vi "Write Non-Sequential Address.vi"(7 "Target IC (1-8)":u8, 8 "error in (no error)":errorcluster, 9 "Data":u16 format="%04x", 10 "Address":u16 format="%04x", 11 "FPGA Interface in":refnum<class "FPGA Interface.lvclass">) -> (0 "error out":errorcluster)   [LabVIEW 2020, in "BCI-1553 API.lvlib" / "FPGA Interface.lvlib" / "FPGA Interface.lvclass"]
doc: "Write a value to an arbitrary address on a component in the 1553 Session."
uses:
  FPGA Interface.lvclass
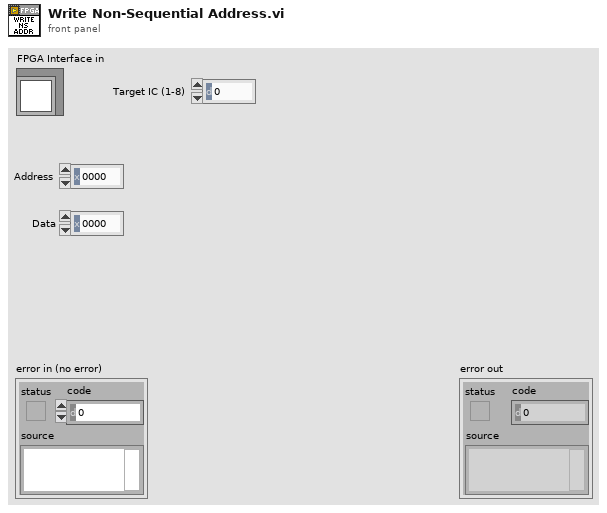
[diagram p1: front panel]
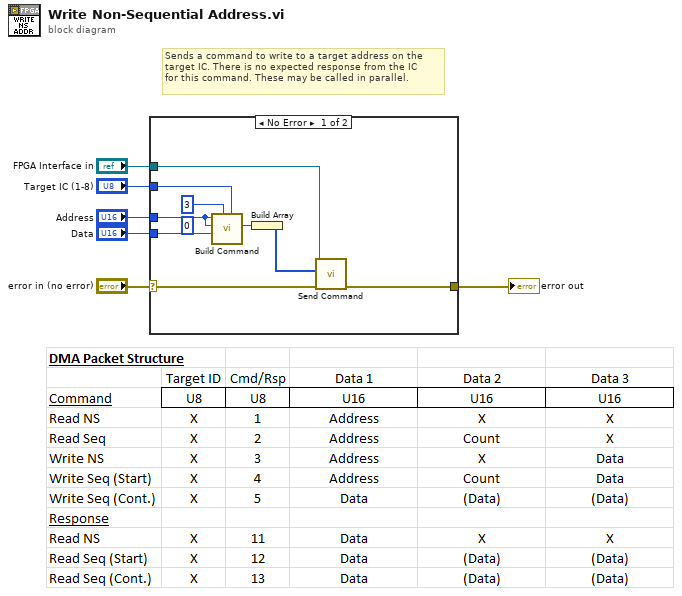
[diagram p0: block diagram]
diagram:
  # "Sends a command to write to a target address on the\ntarget IC. There is no expected response from the IC\nfor this command. These may be called in parallel."
  n1 = case shown="No Error" "error in (no error)" {
    selector: "error in (no error)" -> [w10 w16]
    tunnel: [w9 w16] -> w5
    tunnel: "FPGA Interface in" -> [w12 _]
    tunnel: "Target IC (1-8)" -> [w11 _]
    tunnel: "Address" -> [w7 _]
    tunnel: "Data" -> [w8 _]
    frame No Error {
      (unwired) u16 0 ("Data 2")
      n2 = call "Build Command.vi"("Target"=w11, "CMD ID"=u8 3, "Data 3"=w8, "Data 2"=w7, "Data 1"=w7) -> ("Command"=w15:u64)  [unwired: 5 in, 1 out]
      n3 = Build Array(w15) -> (w14:u64[])
      n4 = call "Send Command.vi"("error in (no error)"=w10, "Data"=w14, "FPGA Interface in"=w12) -> ("error out"=w9:errorcluster)  [unwired: 8 in]
    }
    frame Error {
    }
  }
  "error out" <- w5
